vi "Enqueue.vi"(7 "Priority (f)":bool, 8 "ErrorArray":errorcluster[](array[cluster]), 9 "Data":variant, 10 "Msg":string) -> (0 "ErrorArray":errorcluster[](array[cluster]))   [LabVIEW 2014, in "Framework.lvlib"]
uses:
  Framework.lvlib
  <userlib>/NIST/NISTErrorLib/NISTErrorLib.lvlib
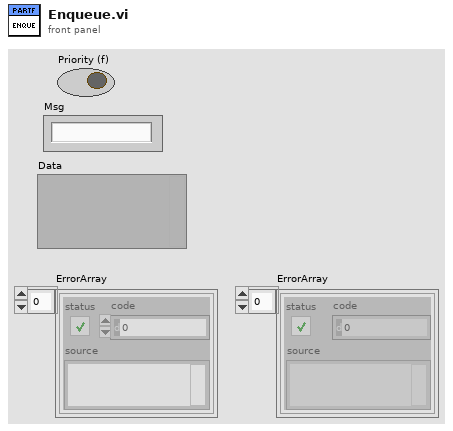
[diagram p1: front panel]
types:
  T1 = typedef "Framework.lvlib/QueRef.ctl" = refnum<queue>
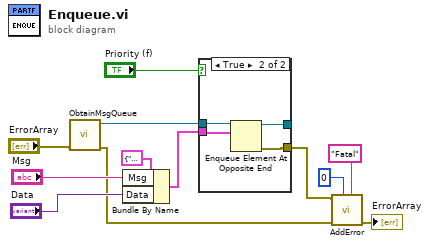
[diagram p0: block diagram]
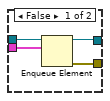
[diagram p2: hidden frame]
diagram:
  n1 = call "ObtainMsgQueue.vi"("ErrorArray"="ErrorArray") -> ("ErrorArray"=w1:errorcluster[], "QueRef"=w3:T1)  [unwired: 9 in]
  n2 = Bundle By Name(cluster=cluster{"Msg":string, "Data":variant} {"Msg"="", "Data"=variant} ("MsgQueue"), "Msg"="Msg", "Data"="Data") -> (w10:cluster{"Msg":string, "Data":variant})
  n3 = case shown="True" "Priority (f)" {
    tunnel: [w13 w20] -> _
    tunnel: w3 -> [w16 w19]
    tunnel: w10 -> [w15 w17]
    tunnel: [w14 w18] -> w7
    frame False {
      n4 = Enqueue Element(queue=w16, element=w15) -> (queue out=w13:T1, error out=w14:errorcluster)  [unwired: 2 in, 1 out]
    }
    frame True {
      n5 = Enqueue Element At Opposite End(queue=w19, element=w17) -> (queue out=w20:T1, error out=w18:errorcluster)  [unwired: 2 in, 1 out]
    }
  }
  n6 = call <userlib>:"AddError.vi"("Severity"="Fatal", "Priority"=u8 0, "ErrorArray"=w1, "error in (no error)"=w7) -> ("ErrorArray"=→"ErrorArray":errorcluster[])  [unwired: 6 in, 1 out]
